vi "BuildRX.vi"() -> (0 "RX":bool[][](array[boolean]))   [LabVIEW 2018]
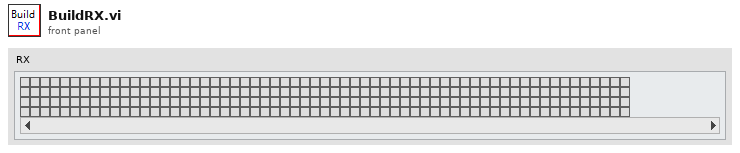
[diagram p1: front panel]
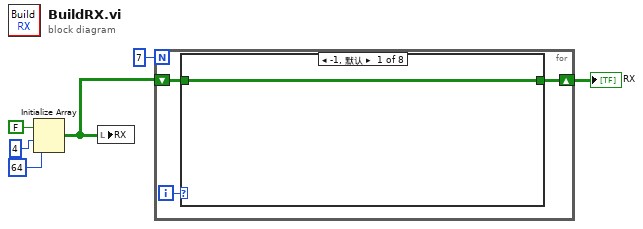
[diagram p0: block diagram]
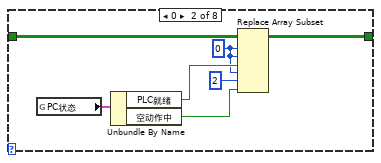
[diagram p2: hidden frame]
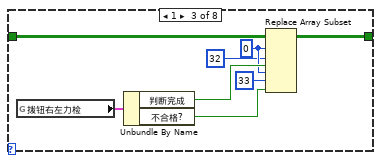
[diagram p3: hidden frame]
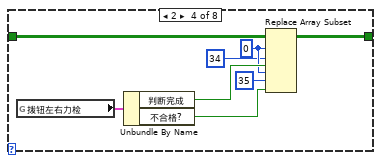
[diagram p4: hidden frame]
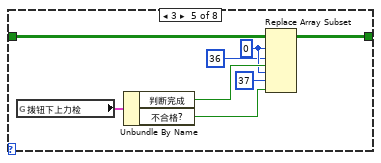
[diagram p5: hidden frame]
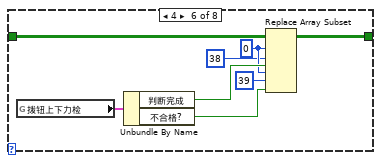
[diagram p6: hidden frame]
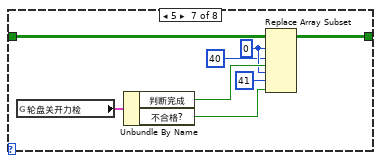
[diagram p7: hidden frame]
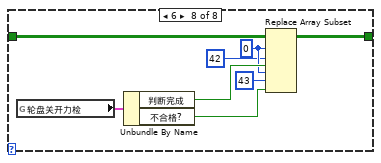
[diagram p8: hidden frame]
diagram:
  n1 = Initialize Array(FALSE, 4 ("维数大小"), 64 ("维数大小")) -> (w6:bool[][])
  n2 = local write "RX"(w6) -> ()
  n3 = for {
    N: 7 -> [_]
    shift-right: [w7] -> w1
    shift-left: w6 -> [w8]
    i -> [w9]
    n4 = case shown="-1, 默认" w9 {
      tunnel: w8 -> [w10 w16 w24 w32 w40 w48 w56 w64]
      tunnel: [w10 w11 w19 w27 w35 w43 w51 w59] -> w7
      frame -1, Default {
      }
      frame 0 {
        w14 = 0 ("索引 (行)")
        n5 = global read "全局 1.vi" "PC状态"() -> (w17:cluster{"PLC就绪":bool, "空动作中":bool})
        n6 = Unbundle By Name(w17) -> ("PLC就绪"=w15:bool, "空动作中"=w12:bool)
        n7 = Replace Array Subset(array=w16, new element #1=w15, index (row) #1=w14, index (col) #1=w14, new element #2=w12, index (row) #2=w14, index (col) #2=2 ("禁用的索引 (列)")) -> (w11:bool[][])
      }
      frame 1 {
        w22 = 0 ("索引 (行)")
        n8 = global read "全局 1.vi" "拨钮右左力检"() -> (w25:cluster{"判断完成":bool, "不合格?":bool})
        n9 = Unbundle By Name(w25) -> ("判断完成"=w23:bool, "不合格?"=w20:bool)
        n10 = Replace Array Subset(array=w24, new element #1=w23, index (row) #1=w22, index (col) #1=32 ("索引 (行)"), new element #2=w20, index (row) #2=w22, index (col) #2=33 ("禁用的索引 (列)")) -> (w19:bool[][])
      }
      frame 2 {
        w30 = 0 ("索引 (行)")
        n11 = global read "全局 1.vi" "拨钮左右力检"() -> (w33:cluster{"判断完成":bool, "不合格?":bool})
        n12 = Unbundle By Name(w33) -> ("判断完成"=w31:bool, "不合格?"=w28:bool)
        n13 = Replace Array Subset(array=w32, new element #1=w31, index (row) #1=w30, index (col) #1=34 ("索引 (行)"), new element #2=w28, index (row) #2=w30, index (col) #2=35 ("禁用的索引 (列)")) -> (w27:bool[][])
      }
      frame 3 {
        w38 = 0 ("索引 (行)")
        n14 = global read "全局 1.vi" "拨钮下上力检"() -> (w41:cluster{"判断完成":bool, "不合格?":bool})
        n15 = Unbundle By Name(w41) -> ("判断完成"=w39:bool, "不合格?"=w36:bool)
        n16 = Replace Array Subset(array=w40, new element #1=w39, index (row) #1=w38, index (col) #1=36 ("索引 (行)"), new element #2=w36, index (row) #2=w38, index (col) #2=37 ("禁用的索引 (列)")) -> (w35:bool[][])
      }
      frame 4 {
        w46 = 0 ("索引 (行)")
        n17 = global read "全局 1.vi" "拨钮上下力检"() -> (w49:cluster{"判断完成":bool, "不合格?":bool})
        n18 = Unbundle By Name(w49) -> ("判断完成"=w47:bool, "不合格?"=w44:bool)
        n19 = Replace Array Subset(array=w48, new element #1=w47, index (row) #1=w46, index (col) #1=38 ("索引 (行)"), new element #2=w44, index (row) #2=w46, index (col) #2=39 ("禁用的索引 (列)")) -> (w43:bool[][])
      }
      frame 5 {
        w54 = 0 ("索引 (行)")
        n20 = global read "全局 1.vi" "轮盘关开力检"() -> (w57:cluster{"判断完成":bool, "不合格?":bool})
        n21 = Unbundle By Name(w57) -> ("判断完成"=w55:bool, "不合格?"=w52:bool)
        n22 = Replace Array Subset(array=w56, new element #1=w55, index (row) #1=w54, index (col) #1=40 ("索引 (行)"), new element #2=w52, index (row) #2=w54, index (col) #2=41 ("禁用的索引 (列)")) -> (w51:bool[][])
      }
      frame 6 {
        w62 = 0 ("索引 (行)")
        n23 = global read "全局 1.vi" "轮盘关开力检"() -> (w65:cluster{"判断完成":bool, "不合格?":bool})
        n24 = Unbundle By Name(w65) -> ("判断完成"=w63:bool, "不合格?"=w60:bool)
        n25 = Replace Array Subset(array=w64, new element #1=w63, index (row) #1=w62, index (col) #1=42 ("索引 (行)"), new element #2=w60, index (row) #2=w62, index (col) #2=43 ("禁用的索引 (列)")) -> (w59:bool[][])
      }
    }
  }
  "RX" <- w1
